vi "DelayCalcMLab.vi"(1 "delay":dbl, 2 "File index number":dbl, 3 "Matrix":sgl[][](array[numeric]), 4 "Sampling Rate":dbl=1000000000.0, 5 "Focal lengths":dbl[](array[numeric])=[0.0085, 0.009, 0.0095, 0.01, 0.0105, 0.011, 0.0115, 0.012, 0.0125, 0.013, 0.0135, 0.014, 0.0145, 0.015], 6 "attn_dB":dbl, 7 "Radii":dbl[](array[numeric])=[0.0, 0.00132, 0.00142, 0.0019, 0.002, 0.00236, 0.00245, 0.00275, 0.00285, 0.0031]) -> (0 "rfnew":sgl[][](array[numeric]))   [LabVIEW 2022 SP3]
panel:
  out "error out":errorcluster
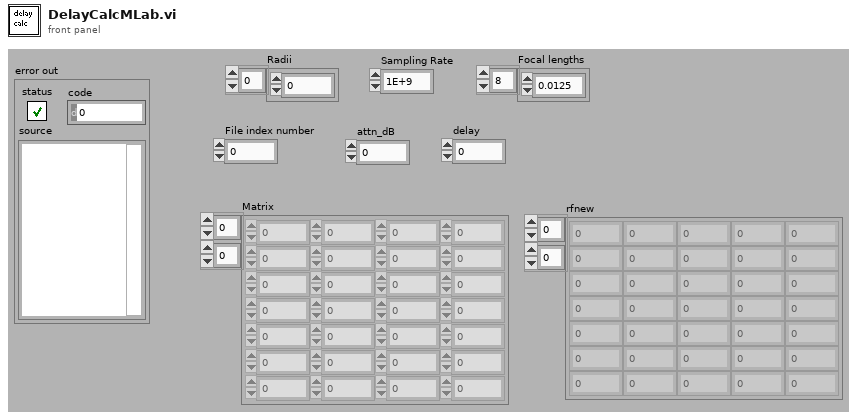
[diagram p1: front panel]
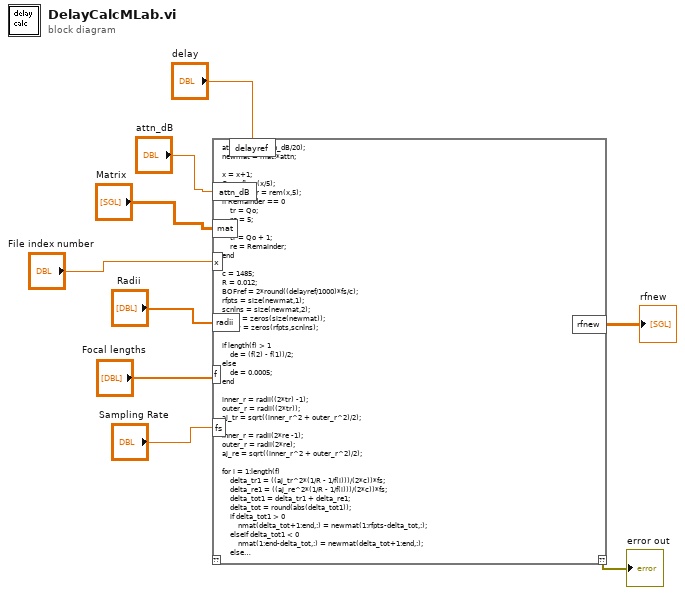
[diagram p0: block diagram]
diagram:
  n1 = script code="attn = 10^(attn_dB/20);\nnewmat = mat.*attn;\n\nx = x+1;\nQo = floor(x/5);\nRemainder = rem(x,5);\nif Remainder == 0\n    tr = Qo;\n    re = 5;\nelse\n    tr = Qo + 1;\n    re = Remainder;\nend\n\nc = 1485;\nR = 0.012;\nBOFref = 2*round((delayref/1000)*fs/c);\nrfpts = size(newmat,1);\nscnlns = size(newmat,2);\nnmat = zeros(size(newmat));\nrfnew = zeros(rfpts,scnlns);\n\nif length(f) > 1\n    de = (f(2) - f(1))/2;\nelse\n    de = 0.0005;\nend\n\ninner_r = radii((2*tr) -1);\nouter_r = radii((2*tr));\naj_tr = sqrt((inner_r^2 + outer_r^2)/2);\n\ninner_r = radii(2*re -1);\nouter_r = radii(2*re);\naj_re = sqrt((inner_r^2 + outer_r^2)/2);\n\nfor i = 1:length(f)\n    delta_tr1 = ((aj_tr^2*(1/R - 1/f(i)))/(2*c))*fs;\n    delta_re1 = ((aj_re^2*(1/R - 1/f(i)))/(2*c))*fs;\n    delta_tot1 = delta_tr1 + delta_re1;\n    delta_tot = round(abs(delta_tot1));\n    if delta_tot1 > 0\n        nmat(delta_tot+1:end,:) = newmat(1:rfpts-delta_tot,:);\n    elseif delta_tot1 < 0\n        nmat(1:end-delta_tot,:) = newmat(delta_tot+1:end,:);\n    else\n        nmat(:,:) = newmat(:,:);\n    end\n   \n    t1 = round(((f(i) - de)/c)*fs*2) - BOFref;\n    t2 = round(((f(i) + de)/c)*fs*2) - BOFref;\n\n    if t1< 1\n       t1 = 1;\n    end\n    if t2 > rfpts\n       t2 = rfpts;\n    end\n    if i == 1\n       t1 = 1;\n    end\n    if i == length(f)\n       t2 = rfpts;\n    end\n    rfnew(t1:t2,:) = nmat(t1:t2,:);\nend"("mat"="Matrix", "attn_dB"="attn_dB", "x"="File index number", "radii"="Radii", "f"="Focal lengths", "fs"="Sampling Rate", "delayref"="delay") -> ("??"=→"error out":errorcluster, "rfnew"=→"rfnew":dbl[][])  [unwired: 1 out]
